vi "TDMS Write Data.vi"(7 "Fields Array In":T1[](array[typedef]), 8 "error in (no error)":errorcluster, 9 "Test Results (\"\")":string, 10 "Test Run (1)":i32, 11 "TDMS File Ref":refnum<k34>) -> (0 "error out":errorcluster, 3 "TDMS File Ref":refnum<k34>, 4 "Timing (ms)":T4, 5 "Fields Array Out":T1[](array[typedef]))   [LabVIEW 2011]
uses:
  database/Fields/Field Record.ctl
  database/Fields/Field DataTypes.ctl
  database/Fields/Field NextItem.ctl
  TDMS Timing.ctl
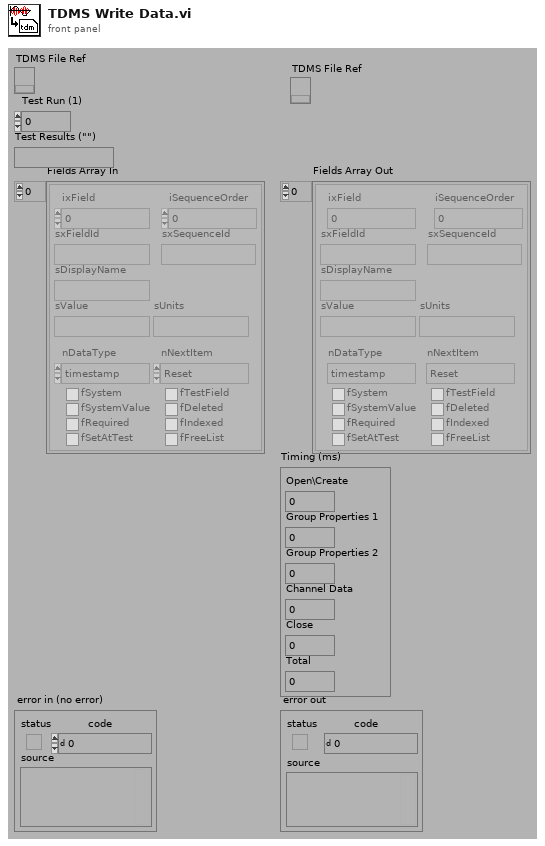
[diagram p1: front panel]
types:
  T1 = typedef "Field Record.ctl" = cluster{"ixField":i32, "iSequenceOrder":i32, "sxFieldId":string, "sxSequenceId":string, "sDisplayName":string, "sValue":string, "sUnits":string, "nDataType":T2, "nNextItem":T3, "fSystem":bool, "fSystemValue":bool, "fRequired":bool, "fSetAtTest":bool, "fTestField":bool, "fDeleted":bool, "fIndexed":bool, "fFreeList":bool}
  T2 = typedef "Field DataTypes.ctl" = enum32{"text", "numeric", "list", "timestamp", "boolean"}
  T3 = typedef "Field NextItem.ctl" = enum32{"Reset", "Retain", "Auto-Increment"}
  T4 = typedef "TDMS Timing.ctl" = cluster{"Open\\Create":u32, "Group Properties 1":u32, "Group Properties 2":u32, "Channel Data":u32, "Close":u32, "Total":u32}
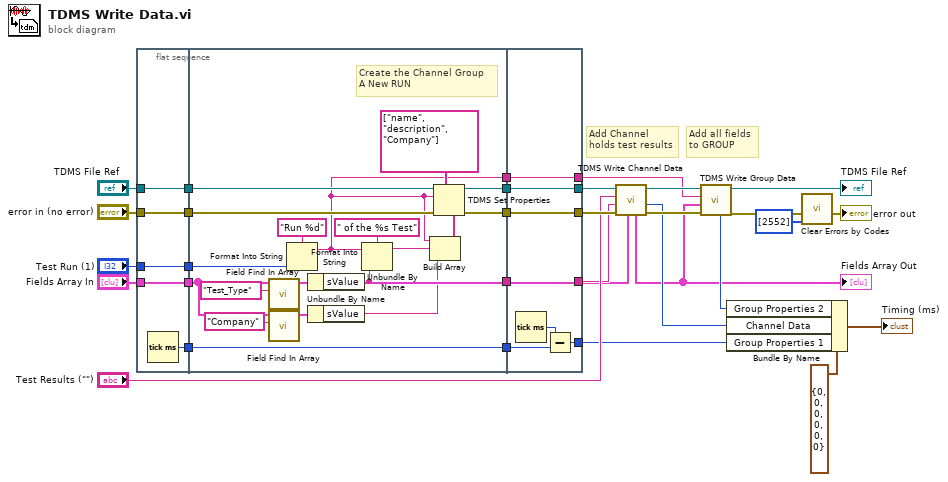
[diagram p0: block diagram]
diagram:
  # "Add Channel\nholds test results"
  # "Add all fields\nto GROUP"
  n1 = flat-sequence {
    tunnel: "Fields Array In" -> [w33]
    tunnel: "error in (no error)" -> [w34]
    tunnel: "TDMS File Ref" -> [w35]
    tunnel: "Test Run (1)" -> [w36]
    tunnel: [w36] -> w19
    tunnel: [w35] -> w18
    tunnel: [w34] -> w17
    tunnel: [w33] -> w16
    tunnel: [w32] -> w14
    tunnel: [w49] -> w22
    tunnel: [w48] -> w21
    tunnel: [w41] -> w20
    tunnel: w19 -> [w53]
    tunnel: w18 -> [w44]
    tunnel: w17 -> [w50]
    tunnel: w16 -> [w37]
    tunnel: [w45] -> w15
    tunnel: w14 -> [w45]
    tunnel: [w42] -> w4
    tunnel: [w60] -> w23
    tunnel: [w61] -> w26
    tunnel: [w62] -> w28
    tunnel: w22 -> [w62]
    tunnel: w21 -> [w61]
    tunnel: w20 -> [w60]
    tunnel: w15 -> [w58]
    tunnel: [w57] -> w11
    tunnel: [w56] -> w5
    tunnel: w4 -> [w56]
    frame #0 {
      n2 = Tick Count (ms)() -> (millisecond timer value=w32:u32)
    }
    frame #1 {
      # "Create the Channel Group\nA New RUN"
      n3 = call "Field Find In Array.vi"("FieldID or Display Name(\"\")"="Test_Type" ("Field Internal ID"), "Field Array"=w37) -> ("Field"=w52:T1)  [unwired: 1 in, 8 out]
      n4 = call "Field Find In Array.vi"("FieldID or Display Name(\"\")"="Company" ("Field_Value"), "Field Array"=w37) -> ("Field"=w39:T1)  [unwired: 1 in, 8 out]
      n5 = Format Into String(format string="Run %d" ("Field Internal ID"), w53) -> (resulting string=w41:string)  [unwired: 2 in, 1 out]
      n6 = Unbundle By Name(w52) -> ("sValue"=w42:string)
      n7 = Unbundle By Name(w39) -> ("sValue"=w38:string)
      n8 = Format Into String(format string=" of the %s Test" ("Field Internal ID"), initial string=w41, w42) -> (resulting string=w46:string)  [unwired: 1 in, 1 out]
      n9 = Build Array(w41, w46, w38) -> (w51:string[])
      n10 = TDMS Set Properties(5:w51, 7:string[] ["name", "description", "Company"], 8:w50, 10:w41, 11:w44) -> (0:w48:errorcluster, 3:w49:refnum<k34>)  [unwired: 3 out]
    }
    frame #2 {
      n11 = Tick Count (ms)() -> (millisecond timer value=w59:u32)
      n12 = Subtract(x=w59, y=w58) -> (x-y=w57:u32)
    }
  }
  n13 = call "TDMS Write Channel Data.vi"("Fields In"="Fields Array In", "error in (no error)"=w26, "Test ID"=w5, "Test Results"="Test Results (\"\")", "TDMS File Ref"=w28) -> ("error out"=w25:errorcluster, "Execution Time (ms)"=w3:u32, "TDMS File Ref"=w27:refnum<k34>, "Fields Out"=w1:T1[])  [unwired: 3 out]
  "Fields Array Out" <- w1
  n14 = call "TDMS Write Group Data.vi"("error in (no error)"=w25, "Fields Array"=w1, "Channel Group"=w23, "TDMS File Ref"=w27) -> ("error out"=w8:errorcluster, "TDMS File Ref"=→"TDMS File Ref":refnum<k34>, "Execution Time (ms)"=w10:u32)  [unwired: 5 out]
  n15 = Bundle By Name(cluster=T4 {"Open\\Create"=0, "Group Properties 1"=0, "Group Properties 2"=0, "Channel Data"=0, "Close"=0, "Total"=0} ("Timing (ms)"), "Group Properties 2"=w10, "Channel Data"=w3, "Group Properties 1"=w11) -> (→"Timing (ms)":T4)
  n16 = call "Clear Errors by Codes.vi"("Error Codes\nto Clear (Empty)"=i32[] [2552] ("Error Codes\nto Clear (Empty)"), "error in (no error)"=w8) -> ("error out"=→"error out":errorcluster)  [unwired: 5 out]
